vi "古田户外一体站流程质控自动启动.vi"(11 "参数":T1={"是否启用仪器"=FALSE, "CODMn"={"启动测量模式"={"测量模式"=enum."水样测量"}, "确定按钮"=TRUE}, "启动模块"={"氨氮1"=FALSE, "总磷1"=FALSE, " COD1"=FALSE}, "常规启动"=FALSE, "直接启动"=FALSE}) -> ()   [LabVIEW 2016, in "质控单元.lvlib"]
uses:
  PLC/PLC.lvlib
panel:
  out "枚举 2":enum16{"初始化", "采配水启动", "等待", "配水", "排水", "结束"}(ring)
  out "枚举":enum16{"初始化", "采配水启动", "等待", "配水", "排水", "结束"}(ring)
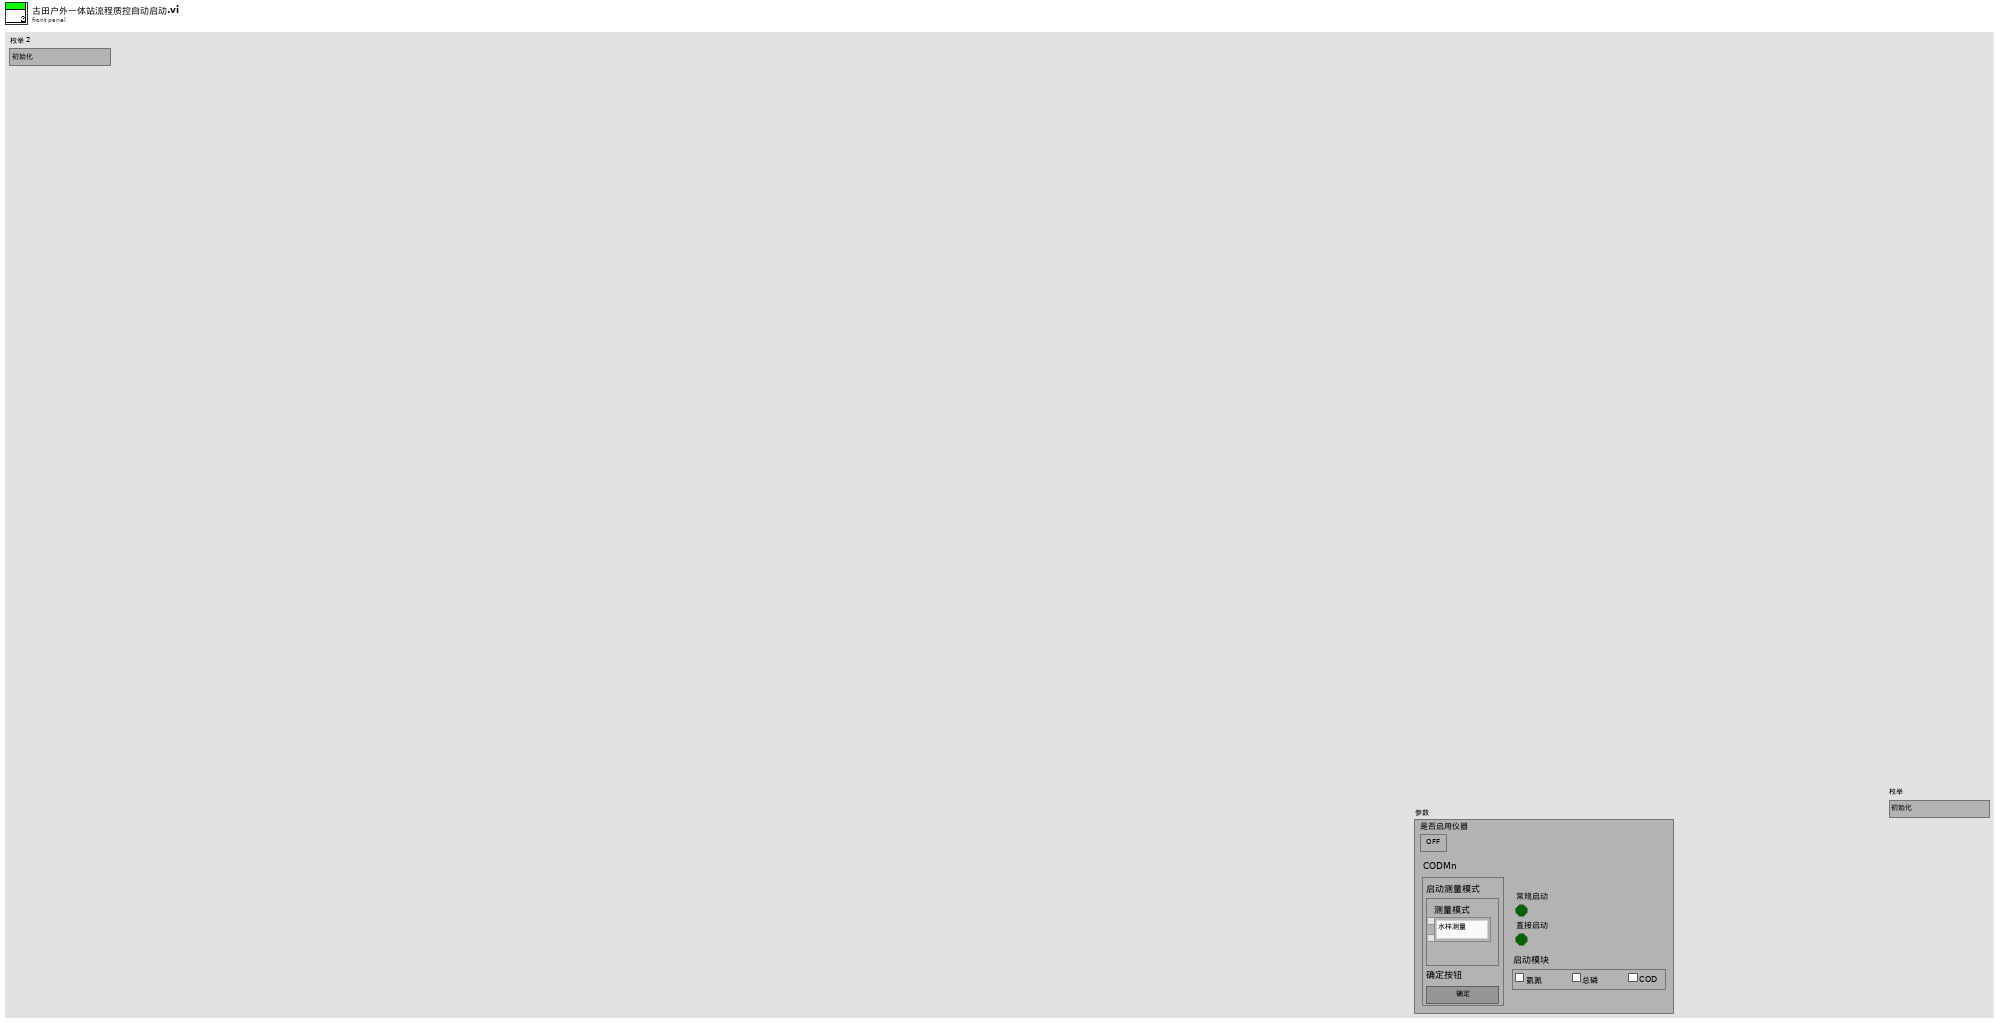
[diagram p1: front panel]
types:
  T1 = cluster{"是否启用仪器":bool, "CODMn":cluster{"启动测量模式":cluster{"测量模式":enum16{"水样测量", "标样核查", "加标回收", "平行样", "校零", "校标"}}, "确定按钮":bool}, "启动模块":cluster{"氨氮1":bool, "总磷1":bool, " COD1":bool}, "常规启动":bool, "直接启动":bool}
  T2 = cluster{"命令":string, cluster{"starting address":u16, "holding register value":u16}}
  T3 = cluster{"R0":i16, "R1":i16, "R2":i16, "R3":i16, "R4":i16, "R5":i16, "R6":i16, "R7":i16, "R8":i16, "R9":i16, "R10":i16, "R11":i16, "R12":i16, "R13":i16, "R14":i16, "R15":i16, "R16":i16, "R17":i16, "R18":i16, "R19":i16}
  T4 = enum32{"Bad", "Idle", "Run top level", "Running"}
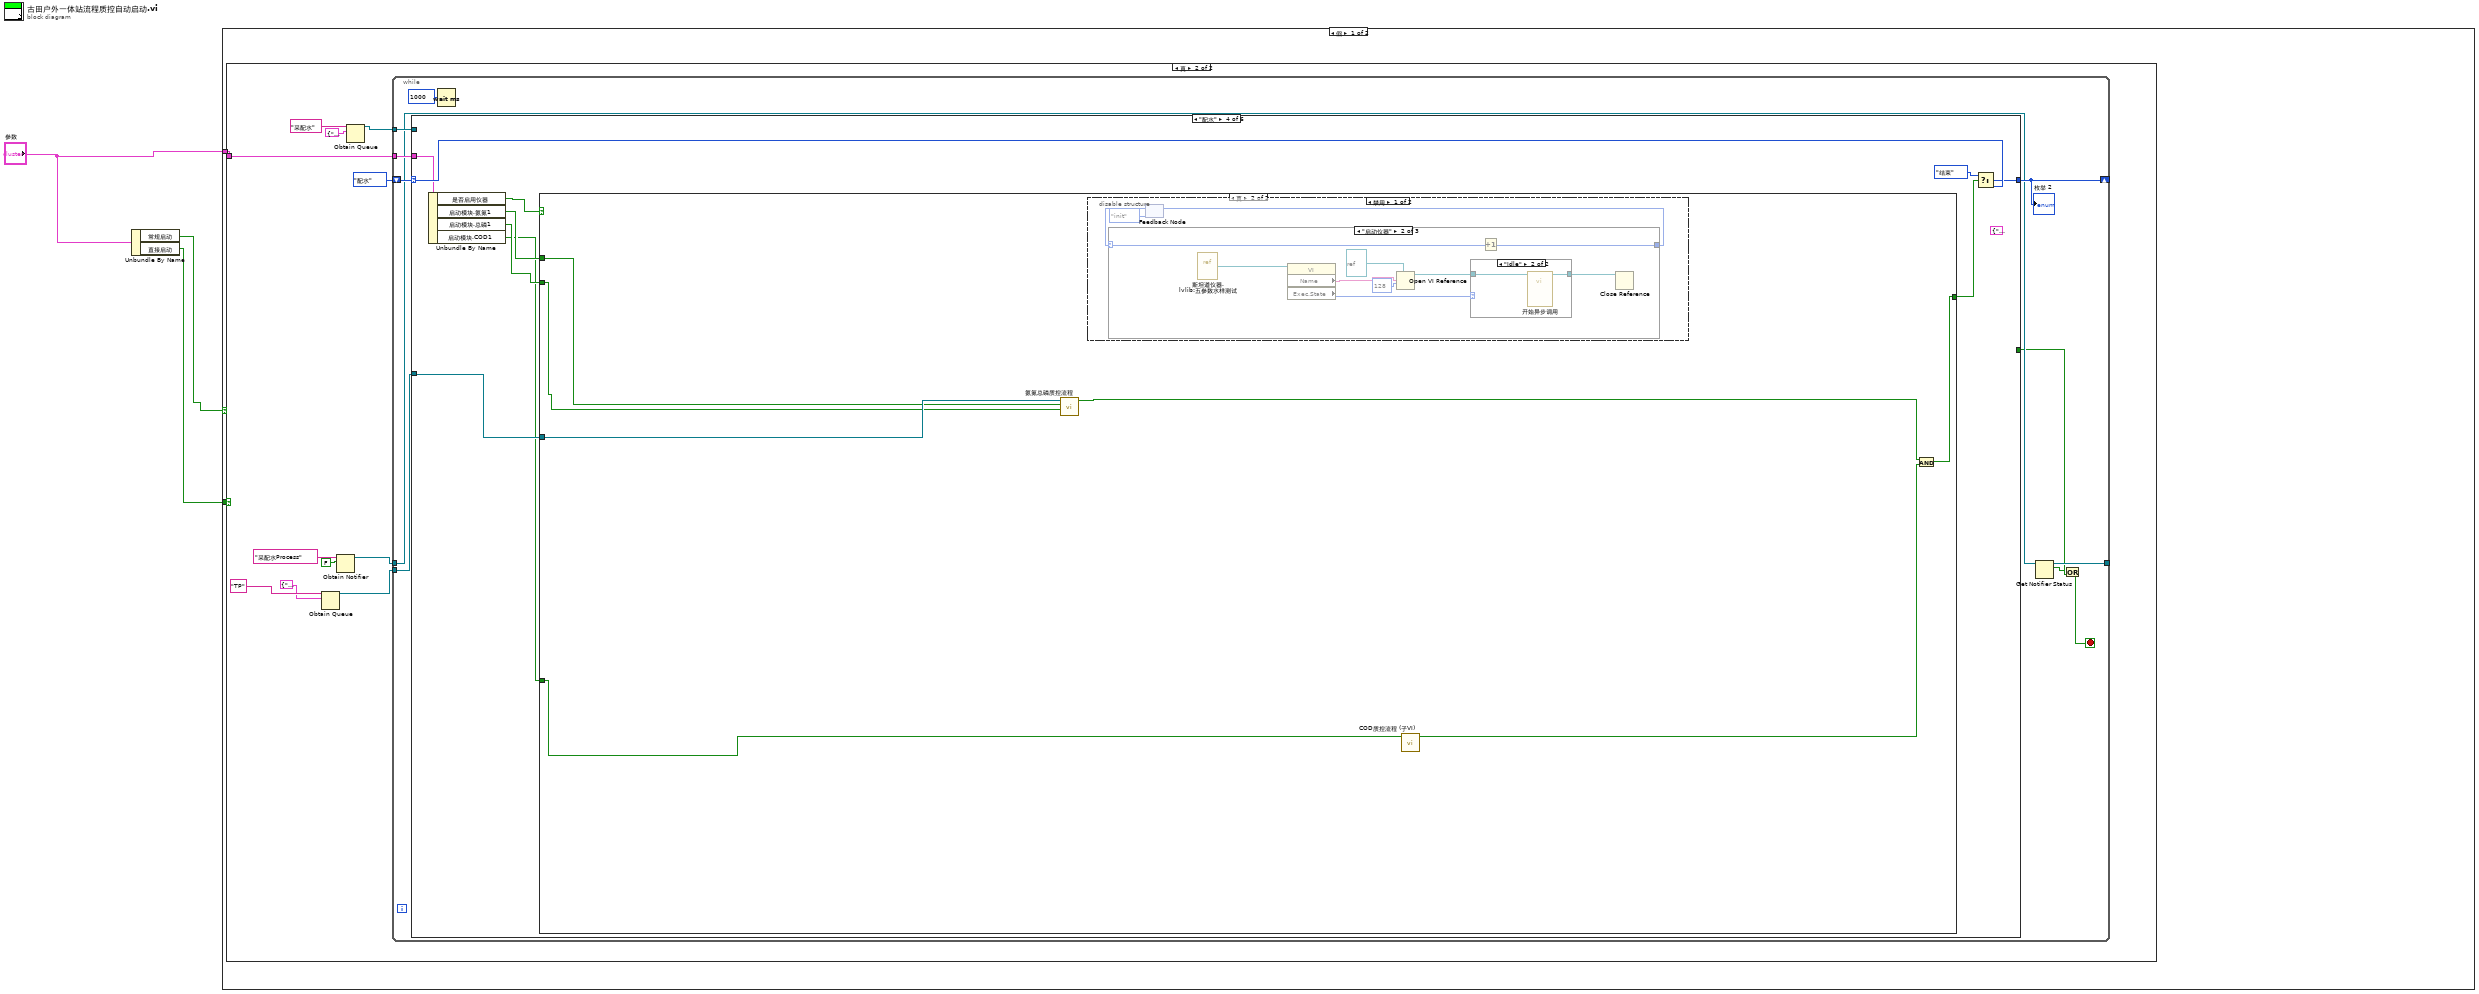
[diagram p0: block diagram]
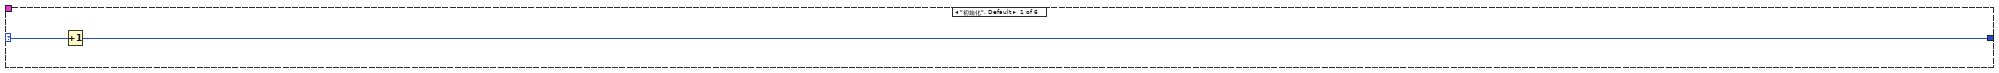
[diagram p3: hidden frame]
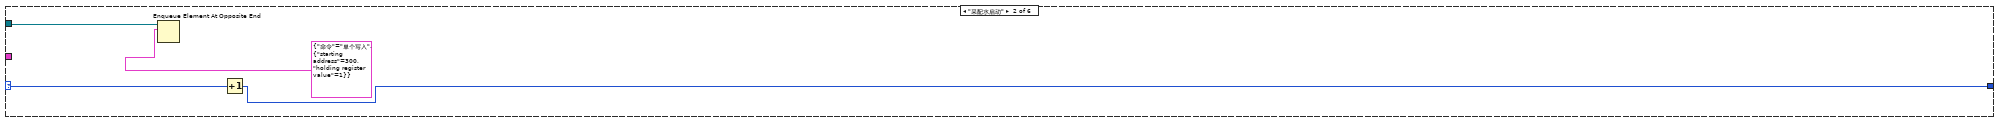
[diagram p4: hidden frame]
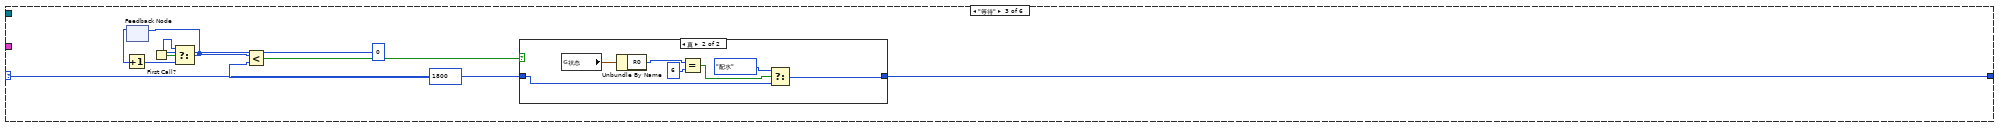
[diagram p5: hidden frame]
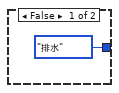
[diagram p6: hidden frame]
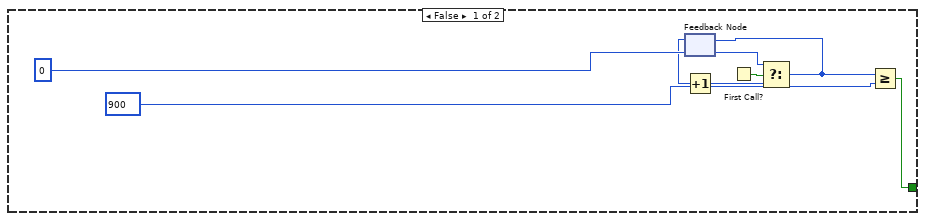
[diagram p7: hidden frame]
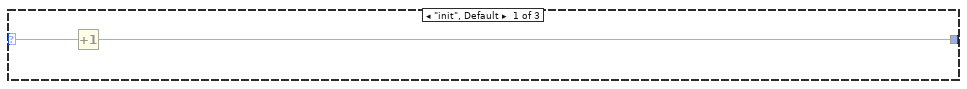
[diagram p8: hidden frame]
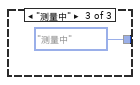
[diagram p10: hidden frame]
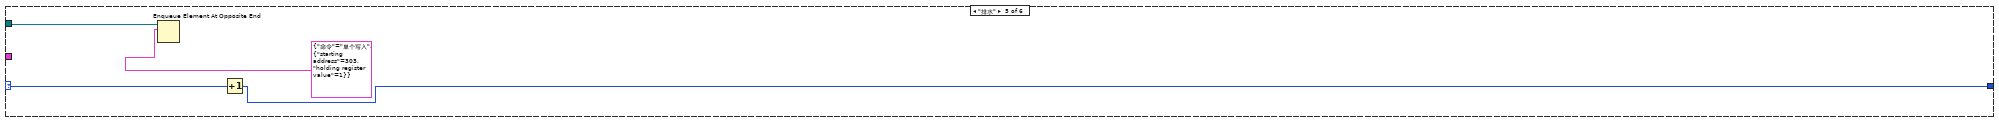
[diagram p12: hidden frame]
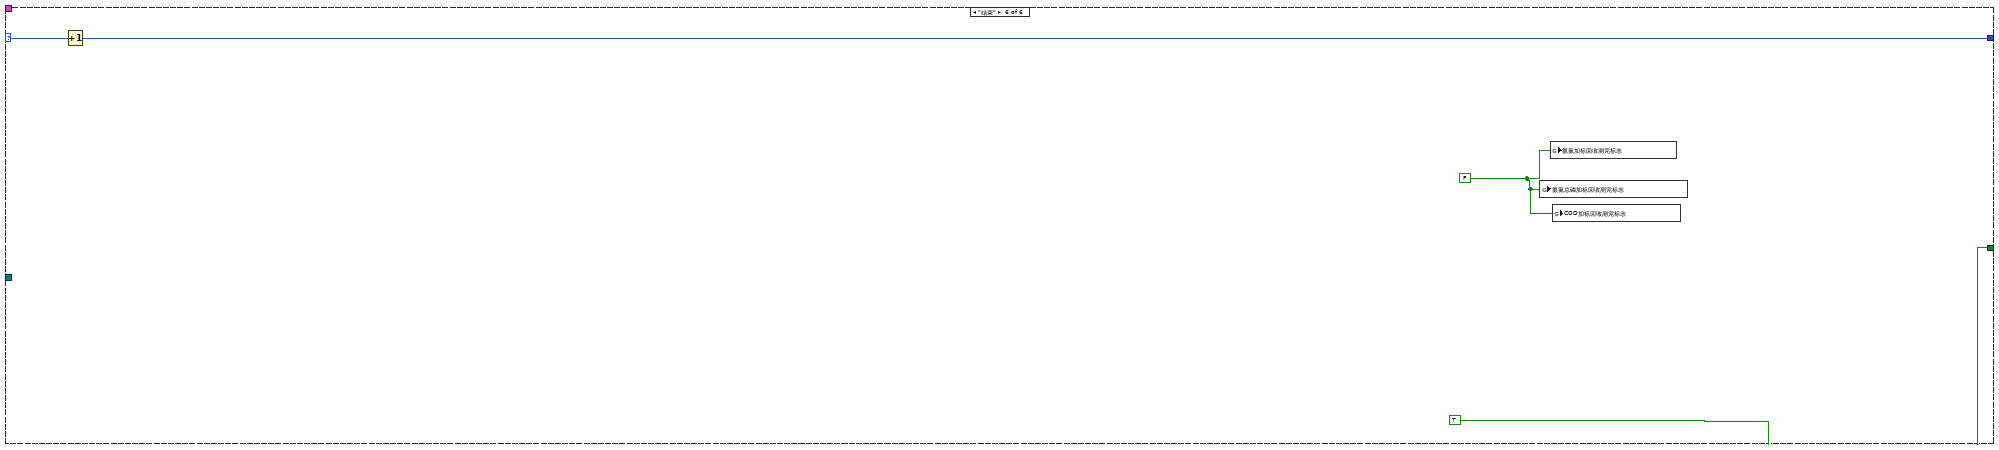
[diagram p13: hidden frame]
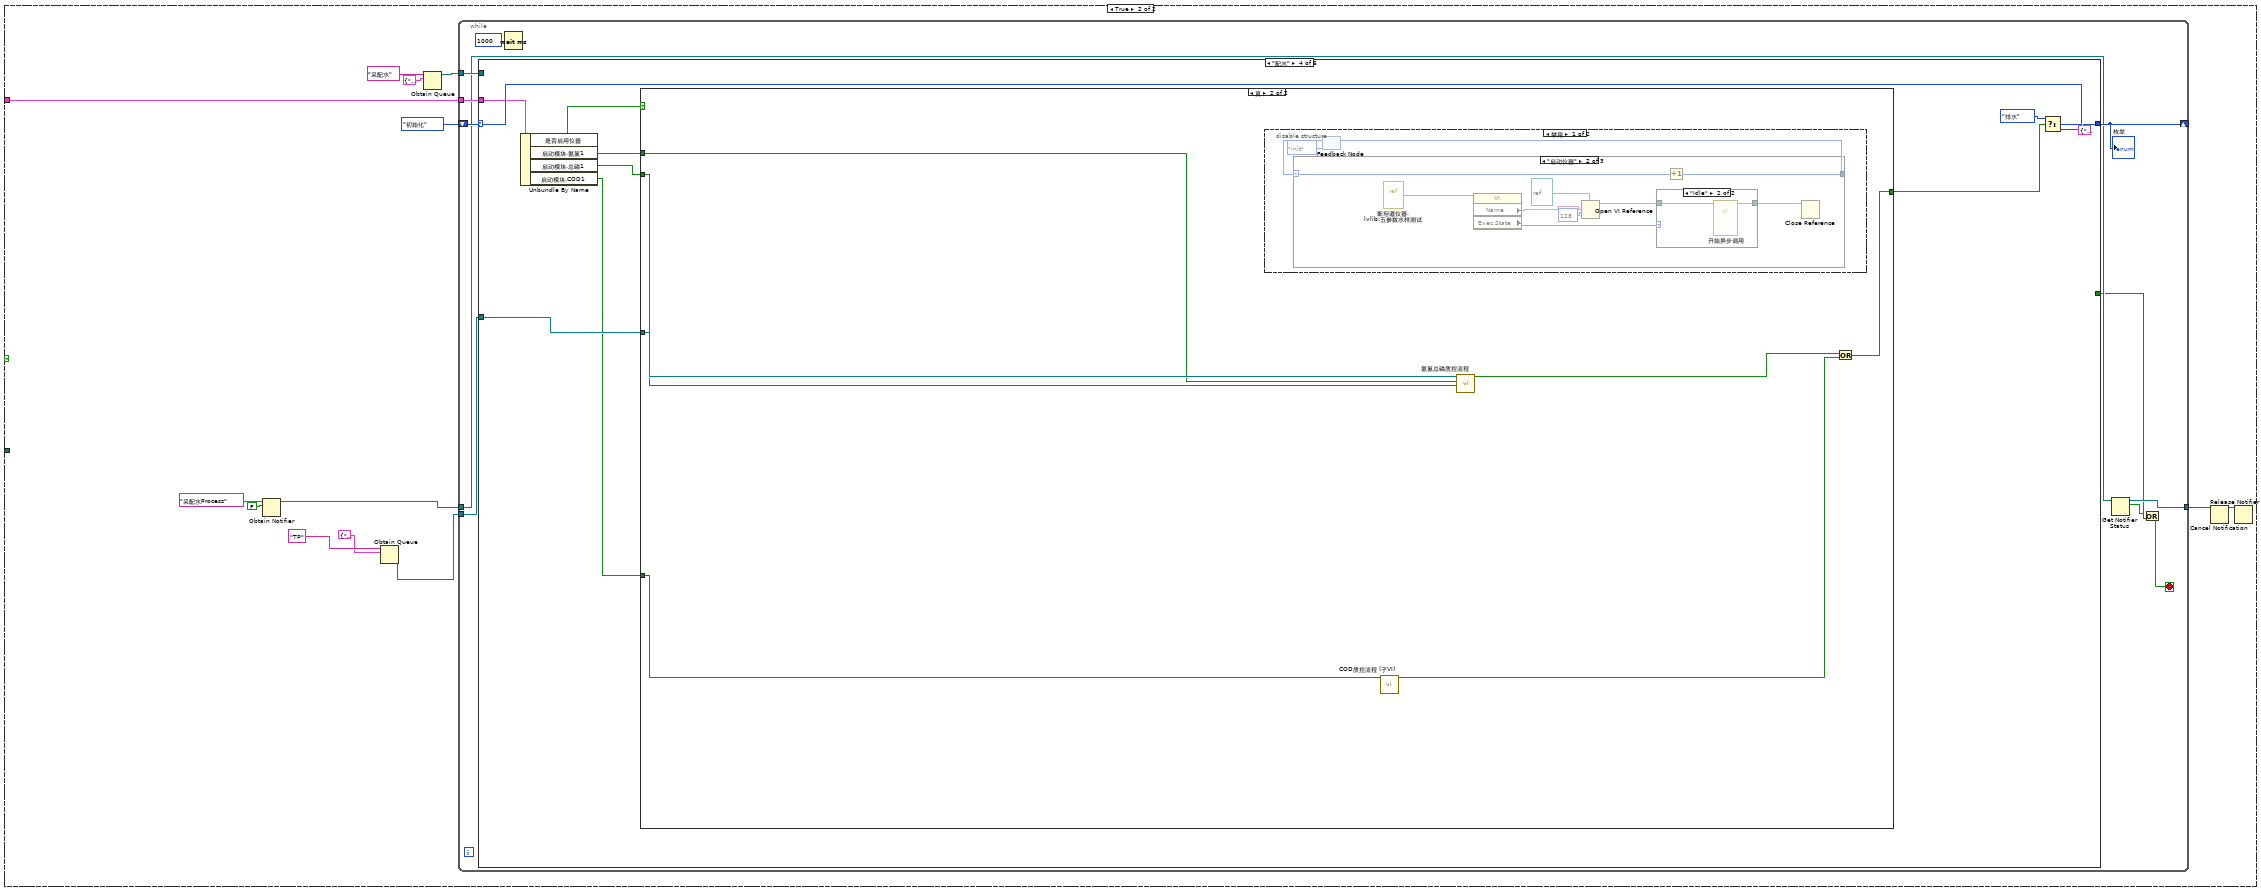
[diagram p14: hidden frame]
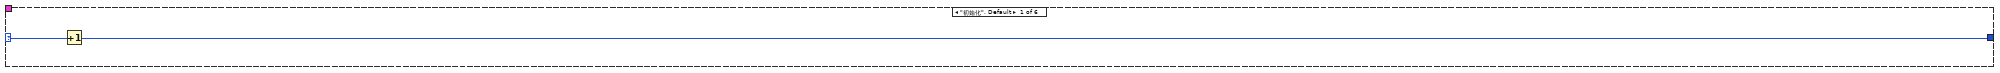
[diagram p15: hidden frame]
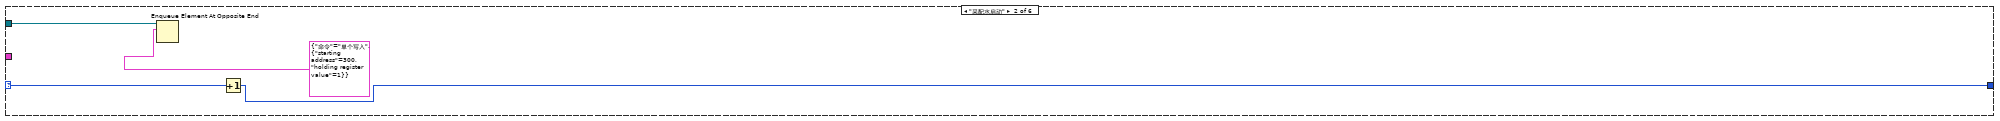
[diagram p16: hidden frame]
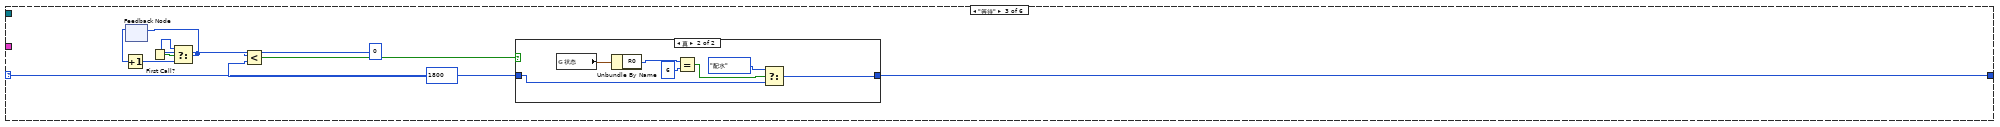
[diagram p17: hidden frame]
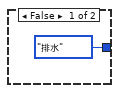
[diagram p18: hidden frame]
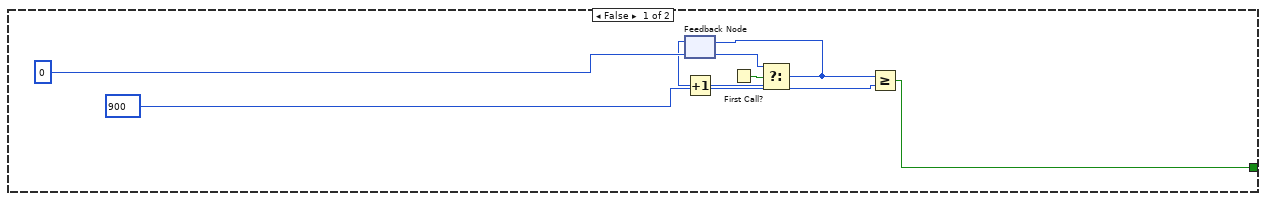
[diagram p19: hidden frame]
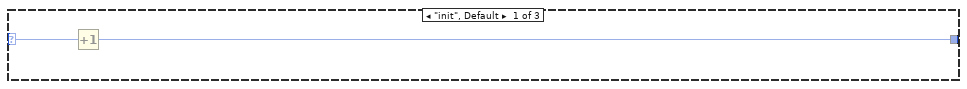
[diagram p20: hidden frame]
diagram:
  n1 = Unbundle By Name("参数") -> ("常规启动"=w2:bool, "直接启动"=w1:bool)
  n2 = case shown="假" w2 {
    tunnel: "参数" -> [w4 w101]
    tunnel: w1 -> [w5 _]
    frame False {
      n3 = case shown="真" w5 {
        tunnel: w4 -> [_ w15]
        frame False {
        }
        frame True {
          n4 = Obtain Queue(name (unnamed)="TP" ("名称（未命名）"), element data type=cluster{"命令":string, "data":variant} {"命令"="", "data"=variant}) -> (queue out=w6:refnum<queue>)  [unwired: 3 in, 2 out]
          n5 = Obtain Notifier(name (unnamed)="采配水Process" ("名称（未命名）"), notification data type=FALSE) -> (notifier out=w9:refnum<notifier>)  [unwired: 2 in, 2 out]
          n6 = Obtain Queue(name (unnamed)="采配水" ("名称（未命名）"), element data type=cluster{"命令":string, "数据":variant} {"命令"="", "数据"=variant}) -> (queue out=w12:refnum<queue>)  [unwired: 3 in, 2 out]
          n7 = while {
            tunnel: w12 -> [w27]
            shift-right: [w25] -> _
            shift-left: enum16{"初始化", "采配水启动", "等待", "配水", "排水", "结束"}."配水" ("枚举") -> [w26]
            tunnel: w6 -> [w23]
            tunnel: w15 -> [w22]
            tunnel: w9 -> [w21]
            tunnel: [w20] -> _
            stop <- w19 stop-if-true
            n8 = case shown="\"配水\"" w26 {
              selector: w26 -> [w29 w31 w40 w59 w94 w100]
              tunnel: w27 -> [_ w32 _ _ w95 _]
              tunnel: [w28 w30 w39 w58 w93 w99] -> w25
              tunnel: [_ _ _ _ _ TRUE] -> w18
              tunnel: w23 -> [_ _ _ w57 _ _]
              tunnel: w22 -> [_ _ _ w54 _ _]
              frame "初始化", Default {
                n9 = Increment(x=w29) -> (x+1=w28:enum16{"初始化", "采配水启动", "等待", "配水", "排水", "结束"})
              }
              frame "采配水启动" {
                n10 = Enqueue Element At Opposite End(queue=w32, element=T2 {"命令"="单个写入", {"starting address"=300, "holding register value"=1}} ("元素")) -> ()  [unwired: 2 in, 3 out]
                n11 = Increment(x=w31) -> (x+1=w30:enum16{"初始化", "采配水启动", "等待", "配水", "排水", "结束"})
              }
              frame "等待" {
                n12 = feedback #1() -> (w36:i32)  [unwired: 1 in]
                n13 = Increment(x=w36) -> (x+1=w35:i32)
                n14 = First Call?() -> (First Call?: T/F=w37:bool)
                n15 = Select(t=0, s=w37, f=w35) -> (s? t:f=w34:i32)
                n16 = feedback-in #1(w34) -> ()
                n17 = Less?(x=w34, y=1800) -> (x < y?=w41:bool)
                n18 = case shown="真" w41 {
                  tunnel: w40 -> [_ w45]
                  tunnel: [enum16{"初始化", "采配水启动", "等待", "配水", "排水", "结束"}."排水" ("枚举") w44] -> w39
                  frame False {
                  }
                  frame True {
                    n19 = global read "采配水全局变量.vi" "状态"() -> (w50:T3)
                    n20 = Unbundle By Name(w50) -> ("R0"=w49:i16)
                    n21 = Equal?(x=w49, y=i16 6) -> (x = y?=w47:bool)
                    n22 = Select(t=enum16{"初始化", "采配水启动", "等待", "配水", "排水", "结束"}."配水" ("枚举"), s=w47, f=w45) -> (s? t:f=w44:enum16{"初始化", "采配水启动", "等待", "配水", "排水", "结束"})
                  }
                }
              }
              frame "配水" {
                (unwired) cluster{"命令":string, "data":variant} {"命令"="启动", "data"=variant(cluster{"站号":u16, "控制命令输出":u16[]} {"站号"=1, "控制命令输出"=[256, 0]})} ("元素")
                n23 = Unbundle By Name(w54) -> ("是否启用仪器"=w56:bool, "启动模块.氨氮1"=w52:bool, "启动模块.总磷1"=w53:bool, "启动模块.COD1"=w51:bool)
                n24 = case shown="真" w56 {
                  tunnel: w57 -> [_ w73]
                  tunnel: [w61 w74] -> w55
                  tunnel: w53 -> [_ w71]
                  tunnel: w52 -> [_ w72]
                  tunnel: w51 -> [_ w70]
                  frame False {
                    n25 = feedback #2() -> (w65:i32)  [unwired: 1 in]
                    n26 = Increment(x=w65) -> (x+1=w64:i32)
                    n27 = First Call?() -> (First Call?: T/F=w66:bool)
                    n28 = Select(t=0, s=w66, f=w64) -> (s? t:f=w62:i32)
                    n29 = feedback-in #2(w62) -> ()
                    n30 = Greater Or Equal?(x=w62, y=900) -> (x >= y?=w61:bool)
                  }
                  frame True {
                    n31 = call "氨氮总磷质控流程.vi"("总磷1"=w71, "氨氮1"=w72, "队列输入"=w73) -> ("布尔"=w68:bool)  [unwired: 8 in]
                    n32 = disable-structure shown="禁用" {
                      frame Disabled {
                        n33 = feedback #3(enum16{"init", "启动仪器", "测量中"}."init") -> (w76:enum16{"init", "启动仪器", "测量中"})
                        n34 = case shown="\"启动仪器\"" w76 {
                          selector: w76 -> [w79 w88 _]
                          tunnel: [w78 w87 enum16{"init", "启动仪器", "测量中"}."测量中"] -> w77
                          frame "init", Default {
                            n35 = Increment(x=w79) -> (x+1=w78:enum16{"init", "启动仪器", "测量中"})
                          }
                          frame "启动仪器" {
                            n36 = vi-ref "斯坦道仪器.lvlib:五参数水样测试.vi"() -> (w80:refnum<vi>)
                            n37 = property class="VI"(reference=w80) -> ("Name"=w84:string, "Exec.State"=w82:T4)  [unwired: 1 in, 2 out]
                            n38 = Open VI Reference(type specifier VI Refnum (for type only)=refnum<vi> refnum ("类型说明符VI引用句柄（仅用于类型）"), vi path=w84, options=128 ("选项")) -> (vi reference=w83:refnum<vi>)  [unwired: 3 in, 1 out]
                            n39 = case shown="\"Idle\"" w82 {
                              tunnel: w83 -> [w89 w91]
                              tunnel: [w89 w90] -> w81
                              frame "Bad", Default {
                              }
                              frame "Idle" {
                                n40 = call-by-ref "开始异步调用"(reference=w91) -> (reference out=w90:refnum<vi>)  [unwired: 13 in, 1 out]
                              }
                            }
                            n41 = Increment(x=w88) -> (x+1=w87:enum16{"init", "启动仪器", "测量中"})
                            n42 = Close Reference(reference=w81) -> ()  [unwired: 1 in, 1 out]
                          }
                          frame "测量中" {
                          }
                        }
                        n43 = feedback-in #3(w77) -> ()
                      }
                      frame Enabled {
                      }
                    }
                    n44 = call "COD质控流程 (子VI).vi"("COD1"=w70) -> ("布尔"=w69:bool)  [unwired: 10 in]
                    n45 = And(x=w68, y=w69) -> (x .and. y?=w74:bool)
                  }
                }
                n46 = Select(t=enum16{"初始化", "采配水启动", "等待", "配水", "排水", "结束"}."结束" ("枚举"), s=w55, f=w59) -> (s? t:f=w58:enum16{"初始化", "采配水启动", "等待", "配水", "排水", "结束"})
              }
              frame "排水" {
                n47 = Enqueue Element At Opposite End(queue=w95, element=T2 {"命令"="单个写入", {"starting address"=303, "holding register value"=1}} ("元素")) -> ()  [unwired: 2 in, 3 out]
                n48 = Increment(x=w94) -> (x+1=w93:enum16{"初始化", "采配水启动", "等待", "配水", "排水", "结束"})
              }
              frame "结束" {
                w97 = FALSE ("氨氮加标回收测完标志")
                n49 = Increment(x=w100) -> (x+1=w99:enum16{"初始化", "采配水启动", "等待", "配水", "排水", "结束"})
                n50 = global write "质控测完标志全局 1.vi" "氨氮总磷加标回收测完标志"(w97) -> ()
                n51 = global write "质控测完标志全局 1.vi" "氨氮加标回收测完标志"(w97) -> ()
                n52 = global write "质控测完标志全局 1.vi" "COD加标回收测完标志"(w97) -> ()
              }
            }
            "枚举 2" <- w25
            n53 = Wait (ms)(milliseconds to wait=u32 1000 ("等待时间（毫秒）")) -> ()  [unwired: 1 out]
            n54 = Get Notifier Status(notifier=w21) -> (notifier out=w20:refnum<notifier>, current notification=w17:bool)  [unwired: 1 in, 3 out]
            n55 = Or(x=w17, y=w18) -> (x .or. y?=w19:bool)
          }
        }
      }
    }
    frame True {
      n56 = Obtain Notifier(name (unnamed)="采配水Process" ("名称（未命名）"), notification data type=FALSE) -> (notifier out=w104:refnum<notifier>)  [unwired: 2 in, 2 out]
      n57 = Obtain Queue(name (unnamed)="TP" ("名称（未命名）"), element data type=cluster{"命令":string, "data":variant} {"命令"="", "data"=variant}) -> (queue out=w107:refnum<queue>)  [unwired: 3 in, 2 out]
      n58 = Obtain Queue(name (unnamed)="采配水" ("名称（未命名）"), element data type=cluster{"命令":string, "数据":variant} {"命令"="", "数据"=variant}) -> (queue out=w111:refnum<queue>)  [unwired: 3 in, 2 out]
      n59 = while {
        tunnel: w111 -> [w124]
        shift-right: [w122] -> _
        shift-left: enum16{"初始化", "采配水启动", "等待", "配水", "排水", "结束"}."初始化" ("枚举") -> [w123]
        tunnel: w107 -> [w120]
        tunnel: w101 -> [w119]
        tunnel: w104 -> [w118]
        tunnel: [w117] -> w103
        stop <- w116 stop-if-true
        n60 = case shown="\"配水\"" w123 {
          selector: w123 -> [w126 w128 w137 w156 w191 w196]
          tunnel: w124 -> [_ w129 _ _ w192 _]
          tunnel: [w125 w127 w136 w155 w190 w195] -> w122
          tunnel: [_ _ _ _ _ TRUE] -> w115
          tunnel: w120 -> [_ _ _ w154 _ _]
          tunnel: w119 -> [_ _ _ w151 _ _]
          frame "初始化", Default {
            n61 = Increment(x=w126) -> (x+1=w125:enum16{"初始化", "采配水启动", "等待", "配水", "排水", "结束"})
          }
          frame "采配水启动" {
            n62 = Enqueue Element At Opposite End(queue=w129, element=T2 {"命令"="单个写入", {"starting address"=300, "holding register value"=1}} ("元素")) -> ()  [unwired: 2 in, 3 out]
            n63 = Increment(x=w128) -> (x+1=w127:enum16{"初始化", "采配水启动", "等待", "配水", "排水", "结束"})
          }
          frame "等待" {
            n64 = feedback #4() -> (w133:i32)  [unwired: 1 in]
            n65 = Increment(x=w133) -> (x+1=w132:i32)
            n66 = First Call?() -> (First Call?: T/F=w134:bool)
            n67 = Select(t=0, s=w134, f=w132) -> (s? t:f=w131:i32)
            n68 = feedback-in #4(w131) -> ()
            n69 = Less?(x=w131, y=1800) -> (x < y?=w138:bool)
            n70 = case shown="真" w138 {
              tunnel: w137 -> [_ w142]
              tunnel: [enum16{"初始化", "采配水启动", "等待", "配水", "排水", "结束"}."排水" ("枚举") w141] -> w136
              frame False {
              }
              frame True {
                n71 = global read "采配水全局变量.vi" "状态"() -> (w147:T3)
                n72 = Unbundle By Name(w147) -> ("R0"=w146:i16)
                n73 = Equal?(x=w146, y=i16 6) -> (x = y?=w144:bool)
                n74 = Select(t=enum16{"初始化", "采配水启动", "等待", "配水", "排水", "结束"}."配水" ("枚举"), s=w144, f=w142) -> (s? t:f=w141:enum16{"初始化", "采配水启动", "等待", "配水", "排水", "结束"})
              }
            }
          }
          frame "配水" {
            (unwired) cluster{"命令":string, "data":variant} {"命令"="启动", "data"=variant(cluster{"站号":u16, "控制命令输出":u16[]} {"站号"=1, "控制命令输出"=[256, 0]})} ("元素")
            n75 = Unbundle By Name(w151) -> ("是否启用仪器"=w153:bool, "启动模块.氨氮1"=w149:bool, "启动模块.总磷1"=w150:bool, "启动模块.COD1"=w148:bool)
            n76 = case shown="真" w153 {
              tunnel: w154 -> [_ w171]
              tunnel: [w158 w168] -> w152
              tunnel: w150 -> [_ w167]
              tunnel: w149 -> [_ w166]
              tunnel: w148 -> [_ w165]
              frame False {
                n77 = feedback #5() -> (w162:i32)  [unwired: 1 in]
                n78 = Increment(x=w162) -> (x+1=w161:i32)
                n79 = First Call?() -> (First Call?: T/F=w163:bool)
                n80 = Select(t=0, s=w163, f=w161) -> (s? t:f=w159:i32)
                n81 = feedback-in #5(w159) -> ()
                n82 = Greater Or Equal?(x=w159, y=900) -> (x >= y?=w158:bool)
              }
              frame True {
                n83 = disable-structure shown="禁用" {
                  frame Disabled {
                    n84 = feedback #6(enum16{"init", "启动仪器", "测量中"}."init") -> (w173:enum16{"init", "启动仪器", "测量中"})
                    n85 = case shown="\"启动仪器\"" w173 {
                      selector: w173 -> [w176 w185 _]
                      tunnel: [w175 w184 enum16{"init", "启动仪器", "测量中"}."测量中"] -> w174
                      frame "init", Default {
                        n86 = Increment(x=w176) -> (x+1=w175:enum16{"init", "启动仪器", "测量中"})
                      }
                      frame "启动仪器" {
                        n87 = vi-ref "斯坦道仪器.lvlib:五参数水样测试.vi"() -> (w177:refnum<vi>)
                        n88 = property class="VI"(reference=w177) -> ("Name"=w181:string, "Exec.State"=w179:T4)  [unwired: 1 in, 2 out]
                        n89 = Open VI Reference(type specifier VI Refnum (for type only)=refnum<vi> refnum ("类型说明符VI引用句柄（仅用于类型）"), vi path=w181, options=128 ("选项")) -> (vi reference=w180:refnum<vi>)  [unwired: 3 in, 1 out]
                        n90 = case shown="\"Idle\"" w179 {
                          tunnel: w180 -> [w186 w188]
                          tunnel: [w186 w187] -> w178
                          frame "Bad", Default {
                          }
                          frame "Idle" {
                            n91 = call-by-ref "开始异步调用"(reference=w188) -> (reference out=w187:refnum<vi>)  [unwired: 13 in, 1 out]
                          }
                        }
                        n92 = Increment(x=w185) -> (x+1=w184:enum16{"init", "启动仪器", "测量中"})
                        n93 = Close Reference(reference=w178) -> ()  [unwired: 1 in, 1 out]
                      }
                      frame "测量中" {
                      }
                    }
                    n94 = feedback-in #6(w174) -> ()
                  }
                  frame Enabled {
                  }
                }
                n95 = call "COD质控流程 (子VI).vi"("COD1"=w165) -> ("布尔"=w169:bool)  [unwired: 10 in]
                n96 = call "氨氮总磷质控流程.vi"("总磷1"=w167, "氨氮1"=w166, "队列输入"=w171) -> ("布尔"=w170:bool)  [unwired: 8 in]
                n97 = Or(x=w170, y=w169) -> (x .or. y?=w168:bool)
              }
            }
            n98 = Select(t=enum16{"初始化", "采配水启动", "等待", "配水", "排水", "结束"}."排水" ("枚举"), s=w152, f=w156) -> (s? t:f=w155:enum16{"初始化", "采配水启动", "等待", "配水", "排水", "结束"})
          }
          frame "排水" {
            n99 = Enqueue Element At Opposite End(queue=w192, element=T2 {"命令"="单个写入", {"starting address"=303, "holding register value"=1}} ("元素")) -> ()  [unwired: 2 in, 3 out]
            n100 = Increment(x=w191) -> (x+1=w190:enum16{"初始化", "采配水启动", "等待", "配水", "排水", "结束"})
          }
          frame "结束" {
            n101 = Increment(x=w196) -> (x+1=w195:enum16{"初始化", "采配水启动", "等待", "配水", "排水", "结束"})
          }
        }
        "枚举" <- w122
        n102 = Wait (ms)(milliseconds to wait=u32 1000 ("等待时间（毫秒）")) -> ()  [unwired: 1 out]
        n103 = Get Notifier Status(notifier=w118) -> (notifier out=w117:refnum<notifier>, current notification=w114:bool)  [unwired: 1 in, 3 out]
        n104 = Or(x=w114, y=w115) -> (x .or. y?=w116:bool)
      }
      n105 = Cancel Notification(0:w103) -> (8:w102:refnum<notifier>)  [unwired: 1 in, 2 out]
      n106 = Release Notifier(notifier=w102) -> ()  [unwired: 2 in, 3 out]
    }
  }
